vi "refresh integration time.vi"(8 "error in (no error)":errorcluster, 11 "LineCCD in":refnum<class "LineCCD.lvclass">) -> (0 "error out":errorcluster, 3 "LineCCD out":refnum<class "LineCCD.lvclass">)   [LabVIEW 2012, in "LineCCD.lvclass"]
uses:
  LineCCD.lvclass
  LineCCD.lvclass/LineCCD.ctl
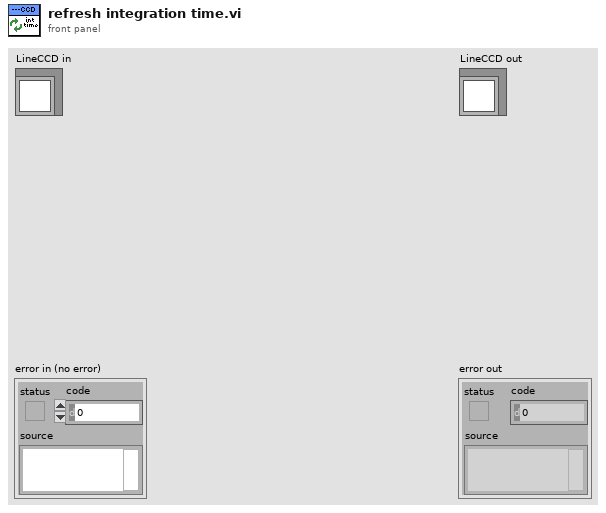
[diagram p1: front panel]
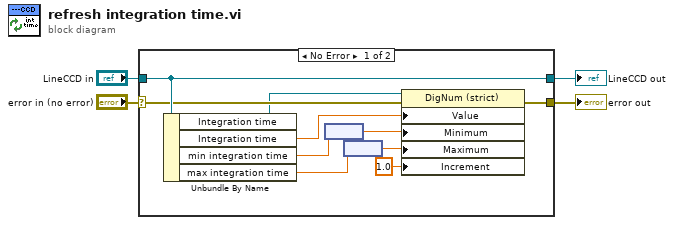
[diagram p0: block diagram]
diagram:
  n1 = case shown="No Error" "error in (no error)" {
    selector: "error in (no error)" -> [w13 w16]
    tunnel: [w12 w16] -> w3
    tunnel: [w14 w15] -> w1
    tunnel: "LineCCD in" -> [w14 w15]
    frame No Error {
      n2 = Unbundle By Name(w14) -> ("Integration time"=w11:refnum<vi>, "Integration time"=w10:dbl[unit], "min integration time"=w9:dbl[unit], "max integration time"=w7:dbl[unit])
      n3 = node(w9) -> (w8:dbl)
      n4 = node(w7) -> (w6:dbl)
      n5 = property class="DigNum (strict)"(reference=w11, error in=w13, "Value"=w10, "Minimum"=w8, "Maximum"=w6, "Increment"=1.0 ("Data Entry Limits:Increment")) -> (error out=w12:errorcluster)  [unwired: 1 out]
    }
    frame Error {
    }
  }
  "error out" <- w3
  "LineCCD out" <- w1
